vi "while_v0_v13.vi"() -> ()   [LabVIEW 2009]
panel:
  out "Contor_w":dbl=15.0
  in  "Latime":dbl(slide)=25.481171548117153 scale=10.0..60.0
  in  "Delay":dbl(slide)=50.04081632653062 scale=10.0..100.0
  out "Waveform Chart":i64(graph)
  in  "stop":bool
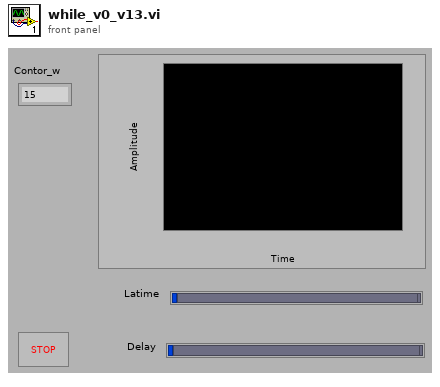
[diagram p1: front panel]
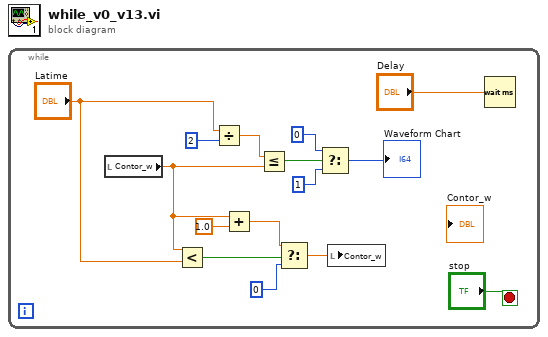
[diagram p0: block diagram]
diagram:
  n1 = while {
    stop <- "stop" stop-if-true
    n2 = local read "Contor_w"() -> (w1:dbl)
    n3 = Less?(x=w1, y="Latime") -> (x < y?=w2:bool)
    n4 = Divide(x="Latime", y=i64 2 ("x")) -> (x/y=w8:dbl)
    n5 = Add(x=w1, y=1.0) -> (x+y=w6:dbl)
    n6 = Less Or Equal?(x=w8, y=w1) -> (x <= y?=w13:bool)
    n7 = Select(t=w6, s=w2, f=0) -> (s? t:f=w5:dbl)
    n8 = Select(t=i64 0, s=w13, f=i64 1) -> (s? t:f=→"Waveform Chart":i64)
    n9 = local write "Contor_w"(w5) -> ()
    n10 = Wait (ms)(milliseconds to wait="Delay") -> ()  [unwired: 1 out]
  }
